vi "GlobalVars.vi"() -> ()   [LabVIEW 2013]
panel:
  in  "Current Position":dbl[](array[numeric])
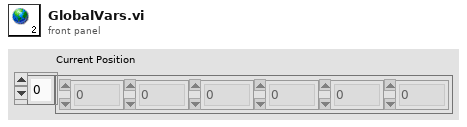
[diagram p1: front panel]
diagram:
